vi "Get Channels.vi"(6 "timeout (ms)":i32=5000, 8 "error in":errorcluster, 11 "gRPC ID":T3) -> (0 "error out":errorcluster, 2 "Channels":T2(array[cluster]), 3 "gRPC ID out":T3)   [LabVIEW 2021, in "CIFCoreWrapper.lvlib"]
uses:
  CIFCoreWrapper.lvlib
  CIFCoreChannel_client/CIFCoreChannel_client.lvlib
  <vilib>/gRPC/LabVIEW gRPC Library/Shared/grpcId.ctl
  <vilib>/gRPC/LabVIEW gRPC Library/grpc-lvsupport-release.lvlib
  CIFCoreChannel_client/RPC Messages/cif_channelcore_Direction.ctl
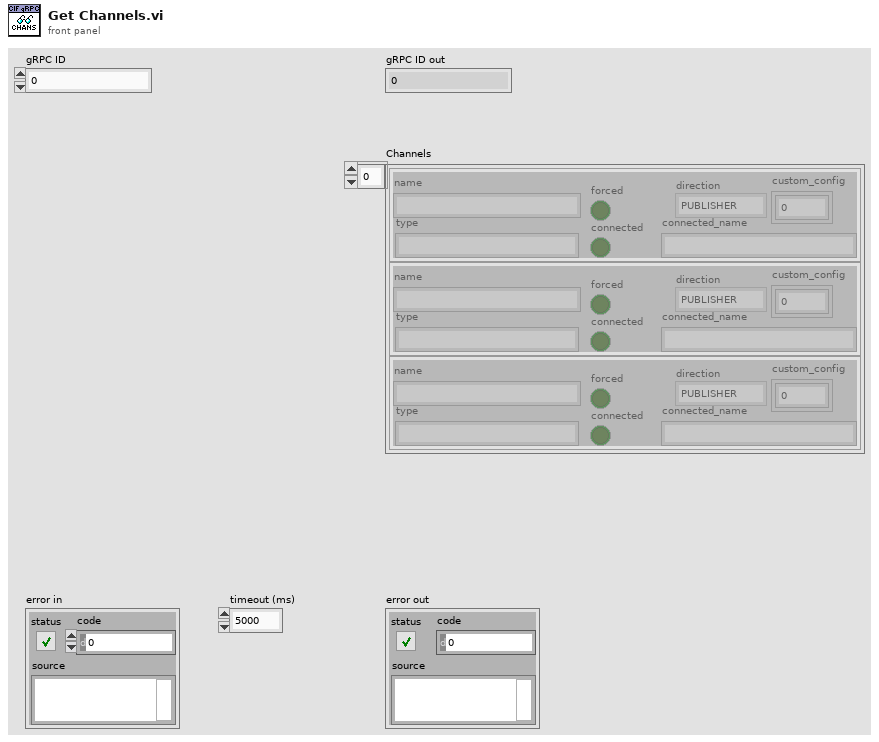
[diagram p1: front panel]
types:
  T1 = typedef "CIFCoreChannel_client.lvlib/cif_channelcore_Direction.ctl" = enum32{"PUBLISHER", "SUBSCRIBER"}
  T2 = cluster{"name":string, "direction":T1, "type":string, "custom_config":u8[], "connected":bool, "connected_name":string, "forced":bool}[]
  T3 = typedef "grpc-lvsupport-release.lvlib/grpcId.ctl" = u64
  T4 = typedef "CIFCoreChannel_client.lvlib/cif_channelcore_Channels.ctl" = cluster{"channels":T5[]}
  T5 = typedef "CIFCoreChannel_client.lvlib/cif_channelcore_Channel.ctl" = cluster{"name":string, "direction":T1, "type":string, "custom_config":u8[], "connected":bool, "connected_name":string, "forced":bool}
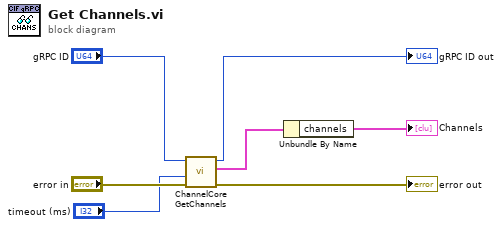
[diagram p0: block diagram]
diagram:
  n1 = call "ChannelCore GetChannels.vi"("error in"="error in", "timeout (ms)"="timeout (ms)", "gRPC ID"="gRPC ID") -> ("error out"=→"error out":errorcluster, "Response Data"=w2:T4, "gRPC ID out"=→"gRPC ID out":T3)  [unwired: 6 in]
  n2 = Unbundle By Name(w2) -> ("channels"=→"Channels":T5[])
